vi "GetSignalParams.vi"(8 "error in (no error)":errorcluster, 11 "FunctionBase in":refnum<class "FunctionBase.lvclass">) -> (0 "error out":errorcluster, 2 "Params":variant, 3 "FunctionBase out":refnum<class "FunctionBase.lvclass">)   [LabVIEW 2018, in "Functions.lvlib" / "FunctionBase.lvclass"]
uses:
  FunctionBase.lvclass
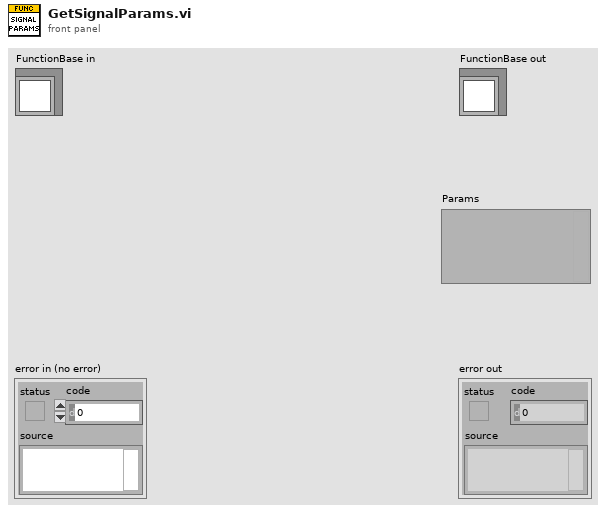
[diagram p1: front panel]
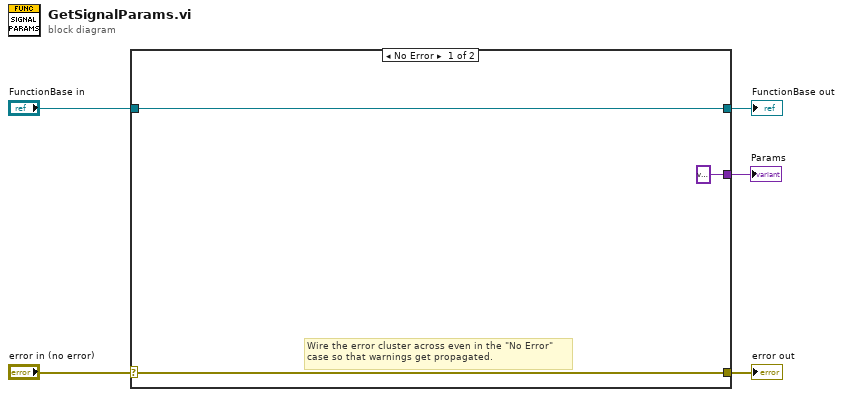
[diagram p0: block diagram]
diagram:
  n1 = case shown="No Error" "error in (no error)" {
    selector: "error in (no error)" -> [w7 w10]
    tunnel: [w7 w10] -> w4
    tunnel: [w8 w9] -> w2
    tunnel: "FunctionBase in" -> [w8 w9]
    tunnel: [variant ("FitterParams") _] -> w1
    frame No Error {
      # "Wire the error cluster across even in the \"No Error\"\ncase so that warnings get propagated."
    }
    frame Error {
    }
  }
  "error out" <- w4
  "FunctionBase out" <- w2
  "Params" <- w1
